vi "NI9205_simpleUI.vi"() -> ()   [LabVIEW 2020]
uses:
  TYPEDEF/NI9205_TD_Method.ctl
panel:
  out "Waveform Graph":waveform(dbl)[](graph)
  in  "Stop":bool
  in  "Start":bool
  in  "Sample Rate":dbl=1000.0
  in  "Number of Samples":i32=100
  in  "Channels NI9205":tag="cDAQ1Mod3/ai0,cDAQ1Mod3/ai2"
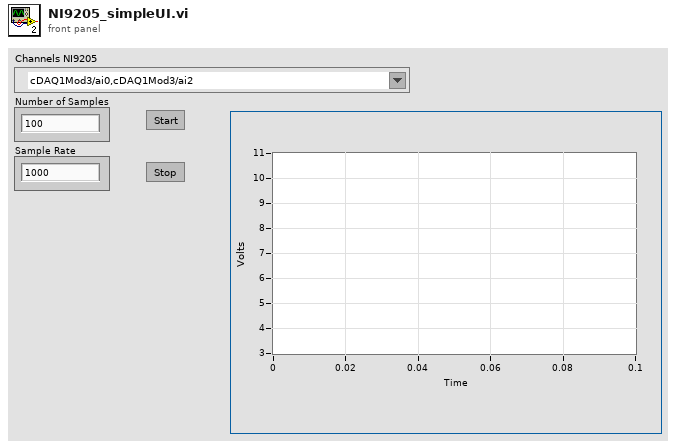
[diagram p1: front panel]
types:
  T1 = typedef "NI9205_TD_Method.ctl" = enum16{"NO_OP", "INIT", "SET", "GET", "CLOSE"}
  T2 = enum8{"Enabled", "Disabled", "Disabled and Grayed Out"}
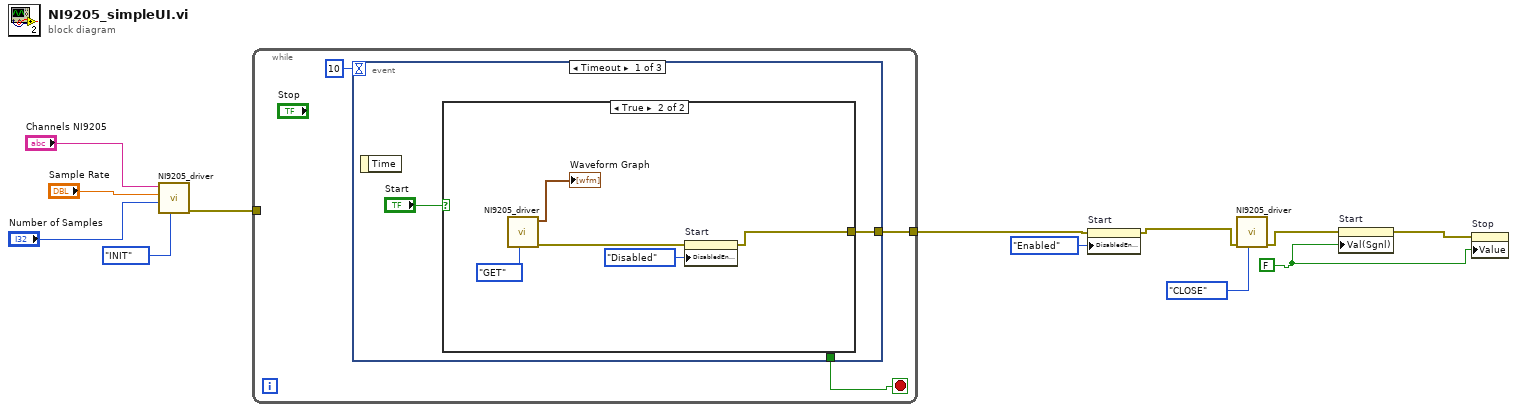
[diagram p0: block diagram]
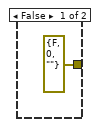
[diagram p2: hidden frame]
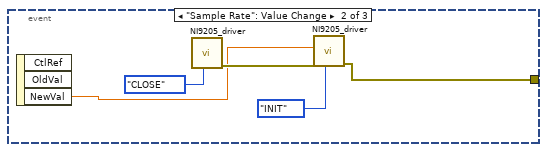
[diagram p3: hidden frame]
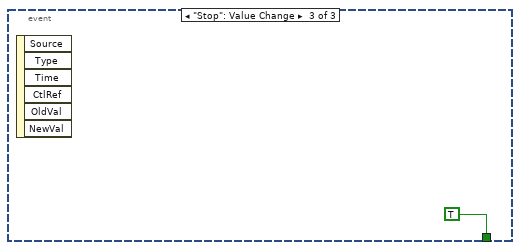
[diagram p4: hidden frame]
diagram:
  w1 = FALSE
  n1 = call "NI9205_driver.vi"("Method NI9205"=NI9205_TD_Method."INIT", "Number of Samples"="Number of Samples", "SampleRate"="Sample Rate", "Channels NI9205"="Channels NI9205") -> ("error out"=w8:errorcluster)  [unwired: 5 in, 2 out]
  n2 = while {
    tunnel: w8 -> [_]
    tunnel: [w15] -> w6
    stop <- w14 stop-if-true
    n3 = event shown="[0] Timeout" {
      selector: _ -> [_ _ _]
      dyn-events: _ -> [_ _ _]
      timeout: 10 -> [_ _ _]
      tunnel: [w16 w24 _] -> w15
      tunnel: [_ _ TRUE] -> w14
      event Timeout {
        n4 = event-data() -> ()  [unwired: 1 in, 1 out]
        n5 = case shown="True" "Start" {
          tunnel: [errorcluster {"status"=FALSE, "code"=0, "source"=""} ("error out") w19] -> w16
          frame False {
          }
          frame True {
            n6 = call "NI9205_driver.vi"("Method NI9205"=NI9205_TD_Method."GET") -> ("error out"=w21:errorcluster, "Waveform Graph"=→"Waveform Graph":waveform(dbl)[])  [unwired: 8 in, 1 out]
            n7 = property on="Start" class="Bool (strict)"(error in=w21, "DisabledEnum"=T2."Disabled" ("Disabled")) -> (error out=w19:errorcluster)  [unwired: 1 in, 1 out]
          }
        }
      }
      event "Sample Rate": Value Change {
        n8 = event-data() -> ("NewVal"=w25:dbl)  [unwired: 1 in, 2 out]
        n9 = call "NI9205_driver.vi"("Method NI9205"=NI9205_TD_Method."CLOSE") -> ("error out"=w26:errorcluster)  [unwired: 8 in, 2 out]
        n10 = call "NI9205_driver.vi"("Method NI9205"=NI9205_TD_Method."INIT", "error in (no error)"=w26, "SampleRate"=w25) -> ("error out"=w24:errorcluster)  [unwired: 6 in, 2 out]
      }
      event "Stop": Value Change {
        n11 = event-data() -> ()  [unwired: 1 in, 6 out]
      }
    }
  }
  n12 = property on="Start" class="Bool (strict)"(error in=w6, "DisabledEnum"=T2."Enabled" ("Disabled")) -> (error out=w4:errorcluster)  [unwired: 1 in, 1 out]
  n13 = call "NI9205_driver.vi"("Method NI9205"=NI9205_TD_Method."CLOSE", "error in (no error)"=w4) -> ("error out"=w3:errorcluster)  [unwired: 7 in, 2 out]
  n14 = property on="Start" class="Bool (strict)"(error in=w3, "Val(Sgnl)"=w1) -> (error out=w2:errorcluster)  [unwired: 1 in, 1 out]
  n15 = property on="Stop" class="Bool (strict)"(error in=w2, "Value"=w1) -> ()  [unwired: 1 in, 2 out]
